vi "MOV_XY_transform.vi"(6 "error in":errorcluster, 7 "芯片角点坐标":T1={"x1(mm)"=1.0, "y1(mm)"=2.0, "x2(mm)"=1.0, "y2(mm)"=7.487, "x1 index"=0, "y1 index"=0, "x2 index"=0, "y2 index"=0, "Chip_POS"=[], "missing"=[]}, 8 "y index":i32, 9 "x index":i32) -> (0 "error out":errorcluster, 2 "Y当前位置(mm)":dbl, 3 "X当前位置(mm)":dbl, 4 "Y实际坐标数":i32, 5 "X实际坐标数":i32)   [LabVIEW 2013]
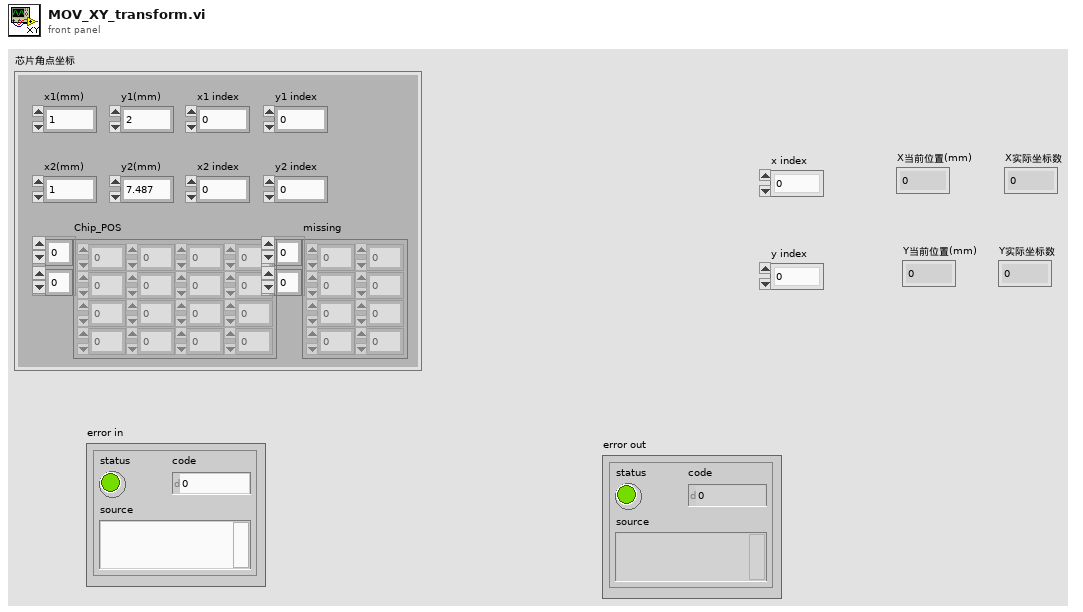
[diagram p1: front panel]
types:
  T1 = cluster{"x1(mm)":dbl, "y1(mm)":dbl, "x2(mm)":dbl, "y2(mm)":dbl, "x1 index":i32, "y1 index":i32, "x2 index":i32, "y2 index":i32, "Chip_POS":dbl[][], "missing":i32[][]}
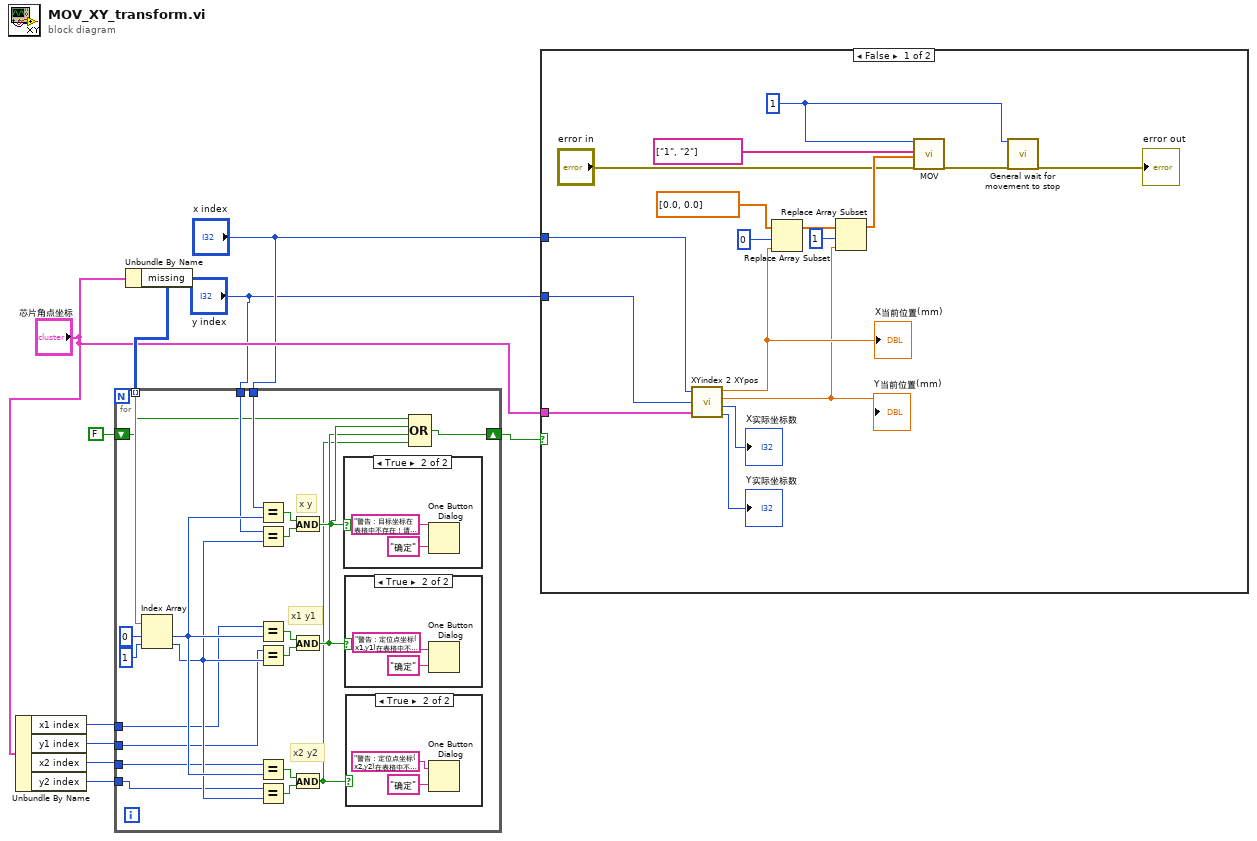
[diagram p0: block diagram]
diagram:
  n1 = Unbundle By Name("芯片角点坐标") -> ("x1 index"=w10:i32, "y1 index"=w8:i32, "x2 index"=w7:i32, "y2 index"=w6:i32)
  n2 = Unbundle By Name("芯片角点坐标") -> ("missing"=w9:i32[][])
  n3 = for {
    tunnel: w9 -> [w32] mode=indexing
    tunnel: "x index" -> [w17]
    tunnel: "y index" -> [w18]
    tunnel: w8 -> [w21]
    tunnel: w10 -> [w20]
    tunnel: w7 -> [w19]
    shift-right: [w16] -> w2
    shift-left: FALSE -> [w15]
    tunnel: w6 -> [w11]
    # "x y"
    # "x2 y2"
    # "x1 y1"
    n4 = Index Array(array=w32, index #1=0 ("索引"), index #2=1 ("索引")) -> (element #1=w23:i32, element #2=w22:i32)
    n5 = Equal?(x=w17, y=w23) -> (x = y?=w29:bool)
    n6 = Equal?(x=w18, y=w22) -> (x = y?=w28:bool)
    n7 = Equal?(x=w20, y=w23) -> (x = y?=w26:bool)
    n8 = Equal?(x=w21, y=w22) -> (x = y?=w27:bool)
    n9 = Equal?(x=w19, y=w23) -> (x = y?=w25:bool)
    n10 = Equal?(x=w11, y=w22) -> (x = y?=w24:bool)
    n11 = And(x=w29, y=w28) -> (x .and. y?=w14:bool)
    n12 = And(x=w26, y=w27) -> (x .and. y?=w13:bool)
    n13 = And(x=w25, y=w24) -> (x .and. y?=w12:bool)
    n14 = case shown="True" w14 {
      frame False {
      }
      frame True {
        n15 = One Button Dialog(message="警告：目标坐标在表格中不存在！请改变目标位置。" ("消息"), button name ("OK")="确定" ("按钮名称（“确定”）")) -> ()  [unwired: 1 out]
      }
    }
    n16 = case shown="True" w13 {
      frame False {
      }
      frame True {
        n17 = One Button Dialog(message="警告：定位点坐标(x1,y1)在表格中不存在！请重新设置。" ("消息"), button name ("OK")="确定" ("按钮名称（“确定”）")) -> ()  [unwired: 1 out]
      }
    }
    n18 = case shown="True" w12 {
      frame False {
      }
      frame True {
        n19 = One Button Dialog(message="警告：定位点坐标(x2,y2)在表格中不存在！请重新设置。" ("消息"), button name ("OK")="确定" ("按钮名称（“确定”）")) -> ()  [unwired: 1 out]
      }
    }
    n20 = Compound Arithmetic op=OR(w15, w14, w13, w12) -> (w16:bool)
  }
  n21 = case shown="False" w2 {
    tunnel: "芯片角点坐标" -> [w42 _]
    tunnel: "x index" -> [w41 _]
    tunnel: "y index" -> [w40 _]
    frame False {
      w45 = 1 ("System no.")
      n22 = call "XYindex 2 XYpos.vi"("x_index"=w41, "y_index"=w40, "芯片角点坐标"=w42) -> ("X当前坐标(mm)"=w47:dbl, "Y当前坐标(mm)"=w46:dbl, "X当前坐标数"=→"X实际坐标数":i32, "Y当前坐标数"=→"Y实际坐标数":i32)
      "X当前位置(mm)" <- w47
      "Y当前位置(mm)" <- w46
      n23 = Replace Array Subset(array=dbl[] [0.0, 0.0], new element=w47, index=0) -> (w52:dbl[])
      n24 = Replace Array Subset(array=w52, new element=w46, index=1) -> (w50:dbl[])
      n25 = call "MOV.vi"("System no."=w45, "Axes to move"=string[] ["1", "2"], "Position values"=w50, "error in"="error in") -> ("error out"=w49:errorcluster)  [unwired: 15 in]
      n26 = call "General wait for movement to stop.vi"("System no."=w45, "error in"=w49) -> ("error out"=→"error out":errorcluster)  [unwired: 16 in, 1 out]
    }
    frame True {
    }
  }
